vi "Listbox-Get Checked Items.vi"(8 "error in (no error)":errorcluster, 11 "reference":refnum<vi>) -> (0 "error out":errorcluster, 3 "Checked Items":string[](array[string]))   [LabVIEW 2020]
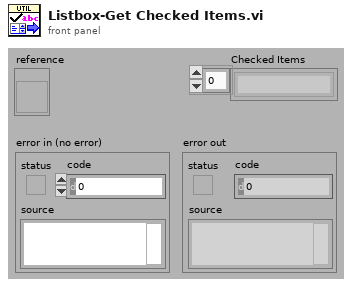
[diagram p1: front panel]
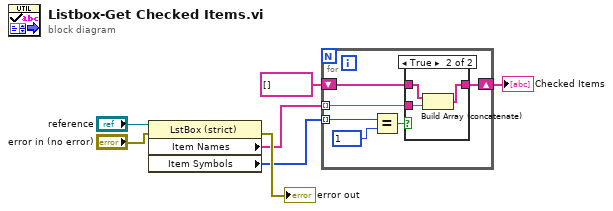
[diagram p0: block diagram]
diagram:
  n1 = property on="Property Node" class="LstBox (strict)"(reference="reference", error in="error in (no error)") -> (error out=→"error out":errorcluster, "Item Names"=w6:string[], "Item Symbols"=w4:i32[])  [unwired: 1 out]
  n2 = for {
    tunnel: w6 -> [w10] mode=indexing
    tunnel: w4 -> [w13] mode=indexing
    shift-right: [w9] -> w1
    shift-left: string[] [] -> [w8]
    n3 = Equal?(x=w13, y=1) -> (x = y?=w11:bool)
    n4 = case shown="True" w11 {
      tunnel: w10 -> [_ w17]
      tunnel: [w14 w16] -> w9
      tunnel: w8 -> [w14 w15]
      frame False {
      }
      frame True {
        n5 = Build Array (concatenate)(w15, w17) -> (w16:string[])
      }
    }
  }
  "Checked Items" <- w1
